vi "Parse String Array.vi"(8 "error in (no error)":errorcluster, 10 "String XYZ":string[][](array[string])) -> (0 "error out":errorcluster, 2 "Line Data":T1)   [LabVIEW 2018, in "Stage Actor.lvlib"]
uses:
  Stage Actor.lvlib
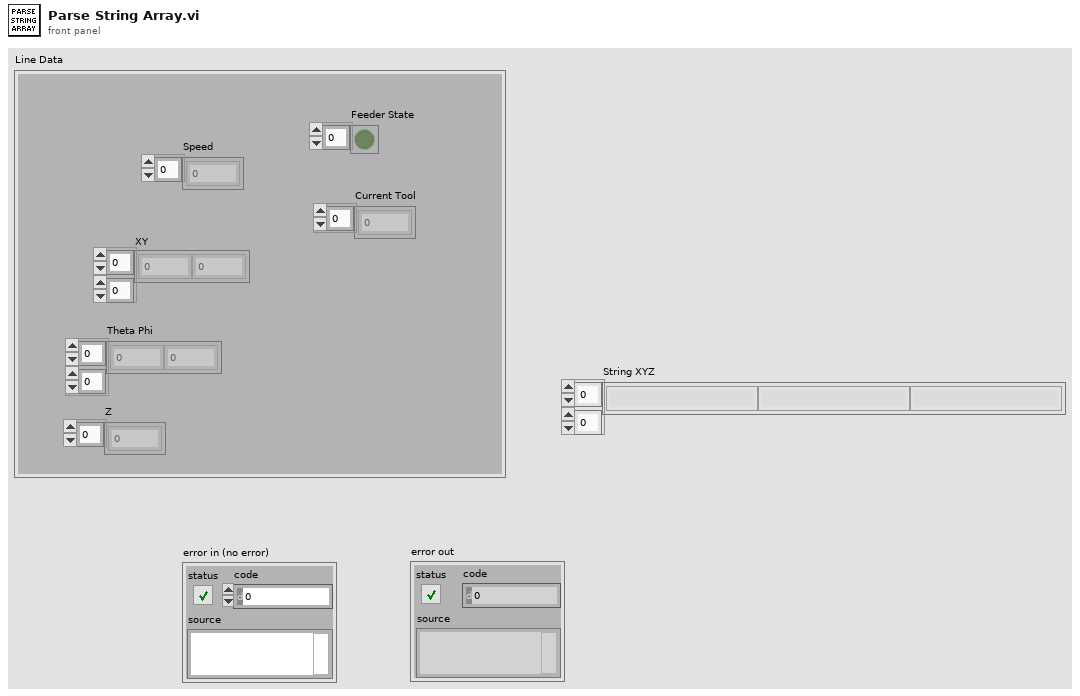
[diagram p1: front panel]
types:
  T1 = cluster{"XY":dbl[][], "Theta Phi":dbl[][], "Current Tool":i16[], "Speed":dbl[], "Feeder State":bool[], "Z":dbl[]}
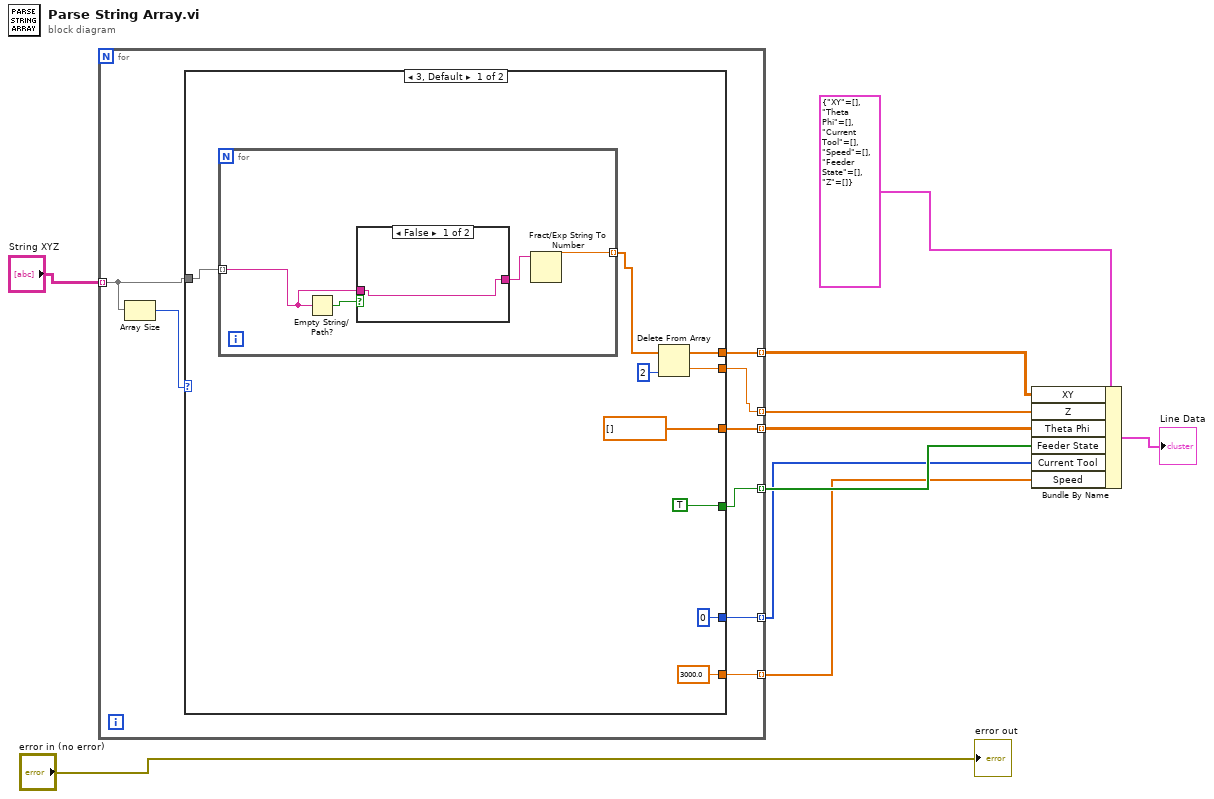
[diagram p0: block diagram]
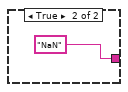
[diagram p2: hidden frame]
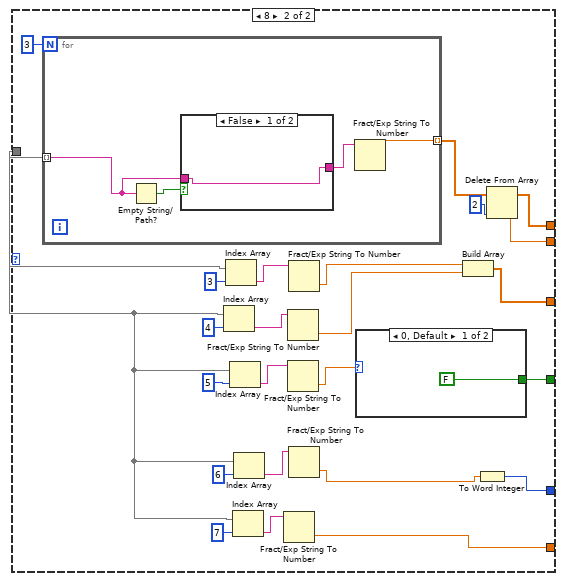
[diagram p3: hidden frame]
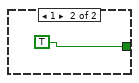
[diagram p4: hidden frame]
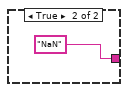
[diagram p5: hidden frame]
diagram:
  n1 = for {
    tunnel: "String XYZ" -> [w14] mode=indexing
    tunnel: [w12] -> w7 mode=indexing
    tunnel: [w18] -> w6 mode=indexing
    tunnel: [w17] -> w5 mode=indexing
    tunnel: [w16] -> w4 mode=indexing
    tunnel: [w15] -> w3 mode=indexing
    tunnel: [w11] -> w1 mode=indexing
    n2 = Array Size(array=w14) -> (size(s)=w13:i32)
    n3 = case shown="3, Default" w13 {
      tunnel: [dbl[] [] w42] -> w18
      tunnel: [TRUE w41] -> w17
      tunnel: [i16 0 w40] -> w16
      tunnel: [3000.0 w39] -> w15
      tunnel: w14 -> [w27 w38]
      tunnel: [w20 w34] -> w12
      tunnel: [w19 w35] -> w11
      frame 3, Default {
        n4 = for {
          tunnel: w27 -> [w30] mode=indexing
          tunnel: [w29] -> w22 mode=indexing
          n5 = Empty String/Path?(string/path=w30) -> (empty?=w31:bool)
          n6 = case shown="False" w31 {
            tunnel: w30 -> [w32 _]
            tunnel: [w32 "NaN" ("String")] -> w28
            frame False {
            }
            frame True {
            }
          }
          n7 = Fract/Exp String To Number(string=w28) -> (number=w29:dbl)  [unwired: 3 in, 1 out]
        }
        n8 = Delete From Array(array=w22, index=2) -> (deleted portion=w20:dbl, array with subset deleted=w19:dbl[])  [unwired: 1 in]
      }
      frame 8 {
        n9 = for {
          N: 3 -> [_]
          tunnel: w38 -> [w62] mode=indexing
          tunnel: [w61] -> w36 mode=indexing
          n10 = Empty String/Path?(string/path=w62) -> (empty?=w63:bool)
          n11 = case shown="False" w63 {
            tunnel: w62 -> [w64 _]
            tunnel: [w64 "NaN" ("String")] -> w60
            frame False {
            }
            frame True {
            }
          }
          n12 = Fract/Exp String To Number(string=w60) -> (number=w61:dbl)  [unwired: 3 in, 1 out]
        }
        n13 = Index Array(array=w38, index=4) -> (element=w45:string)
        n14 = Index Array(array=w38, index=3) -> (element=w46:string)
        n15 = Index Array(array=w38, index=5) -> (element=w55:string)
        n16 = Index Array(array=w38, index=7) -> (element=w50:string)
        n17 = Index Array(array=w38, index=6) -> (element=w51:string)
        n18 = Fract/Exp String To Number(string=w50) -> (number=w39:dbl)  [unwired: 3 in, 1 out]
        n19 = Fract/Exp String To Number(string=w45) -> (number=w44:dbl)  [unwired: 3 in, 1 out]
        n20 = Fract/Exp String To Number(string=w55) -> (number=w54:dbl)  [unwired: 3 in, 1 out]
        n21 = Fract/Exp String To Number(string=w46) -> (number=w43:dbl)  [unwired: 3 in, 1 out]
        n22 = Fract/Exp String To Number(string=w51) -> (number=w49:dbl)  [unwired: 3 in, 1 out]
        n23 = case shown="0, Default" w54 {
          tunnel: [FALSE TRUE] -> w41
          frame 0, Default {
          }
          frame 1 {
          }
        }
        n24 = Build Array(w43, w44) -> (w42:dbl[])
        n25 = To Word Integer(number=w49) -> (16bit integer=w40:i16)
        n26 = Delete From Array(array=w36, index=2) -> (deleted portion=w34:dbl, array with subset deleted=w35:dbl[])  [unwired: 1 in]
      }
    }
  }
  n27 = Bundle By Name(cluster=T1 {"XY"=[], "Theta Phi"=[], "Current Tool"=[], "Speed"=[], "Feeder State"=[], "Z"=[]} ("Line Data 2"), "XY"=w1, "Z"=w7, "Theta Phi"=w6, "Feeder State"=w5, "Current Tool"=w4, "Speed"=w3) -> (→"Line Data":T1)
  "error out" <- "error in (no error)"
